vi "ConfRead.vi"(7 "Section":string, 8 "error in":errorcluster, 9 "type":variant, 10 "key":string="COM", 11 "StructIn":T1) -> (0 "error out":errorcluster, 1 "value":variant, 3 "StructOut":T1)   [LabVIEW 2021, in "LibDan.lvlib"]
uses:
  LibDan.lvlib
  TerminalDef.ctl
  <vilib>/Utility/config.llb/Config Data RefNum.ctl
  <vilib>/Utility/config.llb/Read Key (String).vi
  <vilib>/Utility/config.llb/Read Key (I32).vi
  <vilib>/Utility/config.llb/Read Key (U32).vi
  <vilib>/Utility/config.llb/Read Key (Double).vi
  <vilib>/Utility/Data Type/NI_Data Type.lvlib
  <vilib>/Utility/config.llb/NI_LVConfig.lvlib
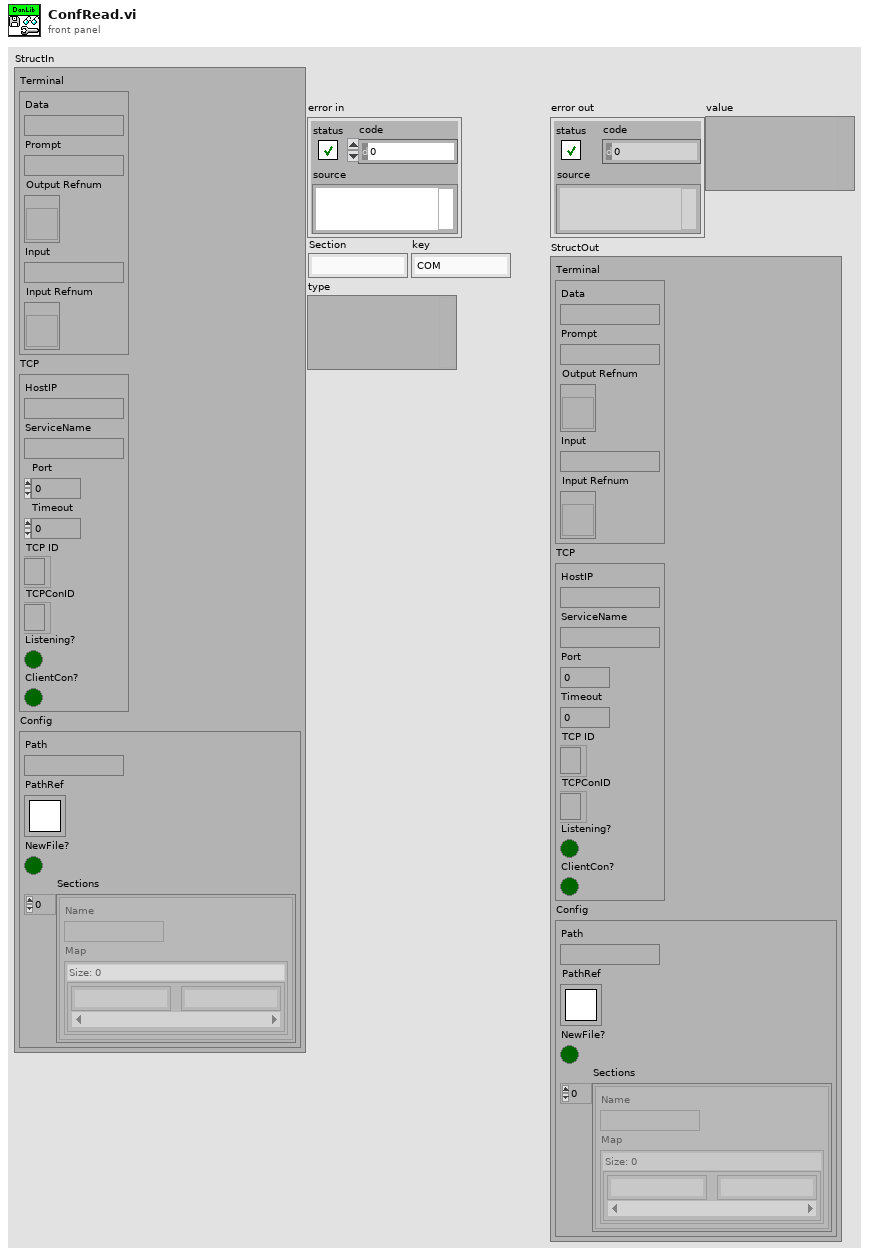
[diagram p1: front panel]
types:
  T1 = typedef "LibDan.lvlib/TerminalDef.ctl" = cluster{"Terminal":cluster{"Data":string, "Prompt":string, "Output Refnum":refnum<vi>, "Input":string, "Input Refnum":refnum<vi>}, "TCP":cluster{"HostIP":string, "ServiceName":string, "Port":u16, "Timeout":i32, "TCP ID":refnum<k5>, "TCPConID":refnum<k5>, "Listening?":bool, "ClientCon?":bool}, "Config":cluster{"Path":path, "PathRef":T2, "NewFile?":bool, "Sections":cluster{"Name":string, "Map":map{string, string}}[]}}
  T2 = typedef "NI_LVConfig.lvlib/Config Data RefNum.ctl" = refnum<k1>
  T3 = cluster{"Name":string, "Map":map{string, string}}[]
  T4 = typedef "NI_Data Type.lvlib/Data Type.ctl" = enum8{"Invalid Type", "Void", "I8", "I16", "I32", "I64", "U8", "U16", "U32", "U64", "Single Float", "Double Float", "Extended Float", "Single Complex", "Double Complex", "Extended Complex", "Enum U8", "Enum U16", "Enum U32", "Enum U64", "Single Float With Unit", "Double Float With Unit", "Extended Float With Unit", "Single Complex with Unit", "Double Complex with Unit", "Extended Complex with Unit", "Boolean", "String", "Path", "Picture", "Tag", "Array", "Cluster", "Variant", "LV Variant", "Waveform", "Timestamp", "Digital Waveform", "Digital Data", "ExpressData", "Refnum", "External Data", "VI", "Poly VI", "LabVIEW Class Instance", "Fixed Point", "Set Collection", "Map Collection"}
  T5 = cluster{"Name":string, "Map":map{string, string}}
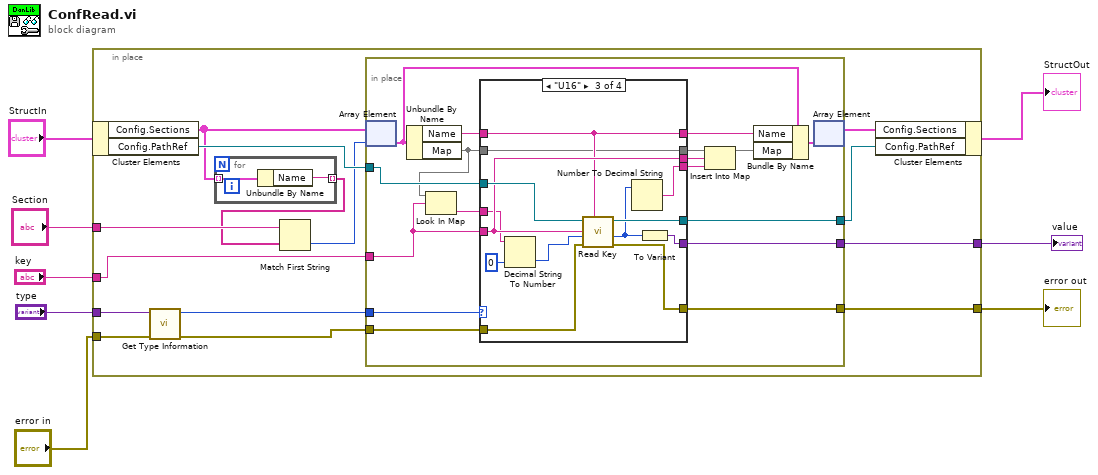
[diagram p0: block diagram]
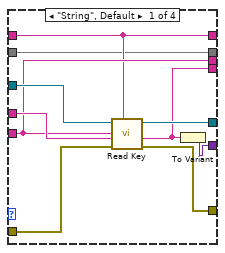
[diagram p2: hidden frame]
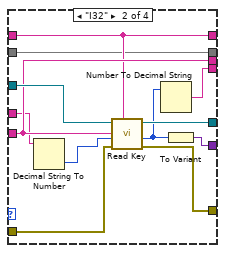
[diagram p3: hidden frame]
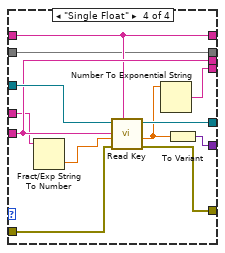
[diagram p4: hidden frame]
diagram:
  n1 = in-place {
    in-place-border: "error in" -> [w15]
    in-place-border: "Section" -> [w21]
    in-place-border: "key" -> [w17]
    in-place-border: "type" -> [w16]
    in-place-border: [w10] -> w2
    in-place-border: [w9] -> w1
    n2 = in-place-cluster #1("StructIn") -> ("Config.Sections"=w20:T3, "Config.PathRef"=w22:T2)
    n3 = call <vilib>:"Get Type Information.vi"("error in (no error)"=w15, "variant"=w16) -> ("error out"=w13:errorcluster, "type"=w14:T4)  [unwired: 5 in, 3 out]
    n4 = for {
      tunnel: w20 -> [w24] mode=indexing
      tunnel: [w23] -> w19 mode=indexing
      n5 = Unbundle By Name(w24) -> ("Name"=w23:string)
    }
    n6 = Match First String(2:w19, 3:w21) -> (0:w18:i32)  [unwired: 1 out]
    n7 = in-place {
      in-place-border: w22 -> [w41]
      in-place-border: w17 -> [w38]
      in-place-border: w14 -> [w40]
      in-place-border: w13 -> [w39]
      in-place-border: [w36] -> w12
      in-place-border: [w26] -> w10
      in-place-border: [w25] -> w9
      n8 = in-place-array #2(w20, w18) -> (w35:T5)
      n9 = Unbundle By Name(w35) -> ("Name"=w34:string, "Map"=w30:map{string, string})
      n10 = Look In Map(map=w30, key=w38) -> (value=w37:string)  [unwired: 1 in, 1 out]
      n11 = case shown="\"U16\"" w40 {
        tunnel: w41 -> [w51 w63 w76 w88]
        tunnel: w39 -> [w49 w62 w75 w87]
        tunnel: w34 -> [w46 w59 w72 w84]
        tunnel: w38 -> [w47 w60 w73 w85]
        tunnel: w37 -> [w50 w56 w69 w81]
        tunnel: [w48 w61 w74 w86] -> w36
        tunnel: [w47 w60 w73 w85] -> w32
        tunnel: [w46 w59 w72 w84] -> w31
        tunnel: [w45 w58 w71 w83] -> w29
        tunnel: w30 -> [w45 w58 w71 w83]
        tunnel: [w42 w54 w67 w79] -> w27
        tunnel: [w44 w57 w70 w82] -> w26
        tunnel: [w43 w52 w65 w77] -> w25
        frame "String", Default {
          n12 = call-poly <vilib>:"Read Key.vi"("section"=w46, "error in (no error)"=w49, "default value"=w50, "key"=w47, "refnum"=w51) -> ("error out"=w44:errorcluster, "value"=w42:string, "refnum out"=w48:T2)  [unwired: 3 in, 1 out]
          n13 = To Variant(anything=w42) -> (Variant=w43:variant)
        }
        frame "I32" {
          n14 = Decimal String To Number(string=w56) -> (number=w55:i32)  [unwired: 2 in, 1 out]
          n15 = call-poly <vilib>:"Read Key.vi"("section"=w59, "error in (no error)"=w62, "default value"=w55, "key"=w60, "refnum"=w63) -> ("error out"=w57:errorcluster, "value"=w53:i32, "refnum out"=w61:T2)  [unwired: 3 in, 1 out]
          n16 = Number To Decimal String(number=w53) -> (decimal integer string=w54:string)  [unwired: 1 in]
          n17 = To Variant(anything=w53) -> (Variant=w52:variant)
        }
        frame "U16" {
          n18 = Decimal String To Number(string=w69, default (0L)=u32 0 ("default (0 I32)")) -> (number=w68:u32)  [unwired: 1 in, 1 out]
          n19 = call-poly <vilib>:"Read Key.vi"("section"=w72, "error in (no error)"=w75, "default value"=w68, "key"=w73, "refnum"=w76) -> ("error out"=w70:errorcluster, "value"=w64:u32, "refnum out"=w74:T2)  [unwired: 3 in, 1 out]
          n20 = Number To Decimal String(number=w64) -> (decimal integer string=w67:string)  [unwired: 1 in]
          n21 = To Variant(anything=w64) -> (Variant=w65:variant)
        }
        frame "Single Float" {
          n22 = Fract/Exp String To Number(string=w81) -> (number=w80:dbl)  [unwired: 3 in, 1 out]
          n23 = call-poly <vilib>:"Read Key.vi"("section"=w84, "error in (no error)"=w87, "default value"=w80, "key"=w85, "refnum"=w88) -> ("error out"=w82:errorcluster, "value"=w78:dbl, "refnum out"=w86:T2)  [unwired: 3 in, 1 out]
          n24 = Number To Exponential String(number=w78) -> (E-format string=w79:string)  [unwired: 3 in]
          n25 = To Variant(anything=w78) -> (Variant=w77:variant)
        }
      }
      n26 = Insert Into Map(map in=w29, key=w32, value=w27) -> (map out=w28:map{string, string})  [unwired: 2 out]
      n27 = Bundle By Name(cluster=w35, "Name"=w31, "Map"=w28) -> (w33:T5)
      n28 = in-place-array #2(w33) -> (w11:T3)  [unwired: 1 out]
    }
    n29 = in-place-cluster #1("Config.Sections"=w11, "Config.PathRef"=w12) -> (→"StructOut":T1)
  }
  "error out" <- w2
  "value" <- w1
